vi "Read All Mixed Module Sizes.vi"(6 "MixedIO Mod Size Idxs":T14, 7 "R/W Case":T13, 8 "error in (no error)":errorcluster, 10 "Async in":T1, 11 "RSI Modules in":T2[](array[typedef]) {"Module Config Data"."Config Block Data Refs"."Data Reference" format="%.0x"; "CDOutput Data"."BD Refs"."Data Reference" format="%.0x"; "CDInput Data"."BD Refs"."Data Reference" format="%.0x"; "VS ref" format="%.0x"}) -> (0 "error out":errorcluster, 2 "Async out":T1, 3 "RSI Modules out":T2[](array[typedef]) {"Module Config Data"."Config Block Data Refs"."Data Reference" format="%.0x"; "CDOutput Data"."BD Refs"."Data Reference" format="%.0x"; "CDInput Data"."BD Refs"."Data Reference" format="%.0x"; "VS ref" format="%.0x"})   [LabVIEW 2020, in "SEECD Engine.lvlib"]
uses:
  SEECD Engine.lvlib
  Type Defs/Mod Size Indexes.ctl
  <vilib>/NI VeriStand/Custom Device API/Custom Device Item Ref.ctl
  <vilib>/NI VeriStand/Custom Device API/Custom Device API.lvlib
  <vilib>/NI VeriStand/Custom Device API/Data Reference.ctl
  <vilib>/NI VeriStand/Custom Device API/Block Data Reference.ctl
  Type Defs/Input Data.ctl
  Type Defs/Output Data.ctl
  Includes/Modules.lvlibp/RSI Module/Channel Type.ctl
  Includes/Modules.lvlibp/RSI Module/RSI Module.lvclass
  Includes/Modules.lvlibp/RSI Module/Module Models.ctl
  Type Defs/Module Config Data.ctl
  Type Defs/Mixed IO.ctl
  Type Defs/Open Module IOVs.ctl
  Type Defs/RSI Module Data.ctl
  Type Defs/RW Case.ctl
  Type Defs/Async Command.ctl
  Type Defs/Async State.ctl
  Type Defs/Async Status.ctl
  Type Defs/Async Data.ctl
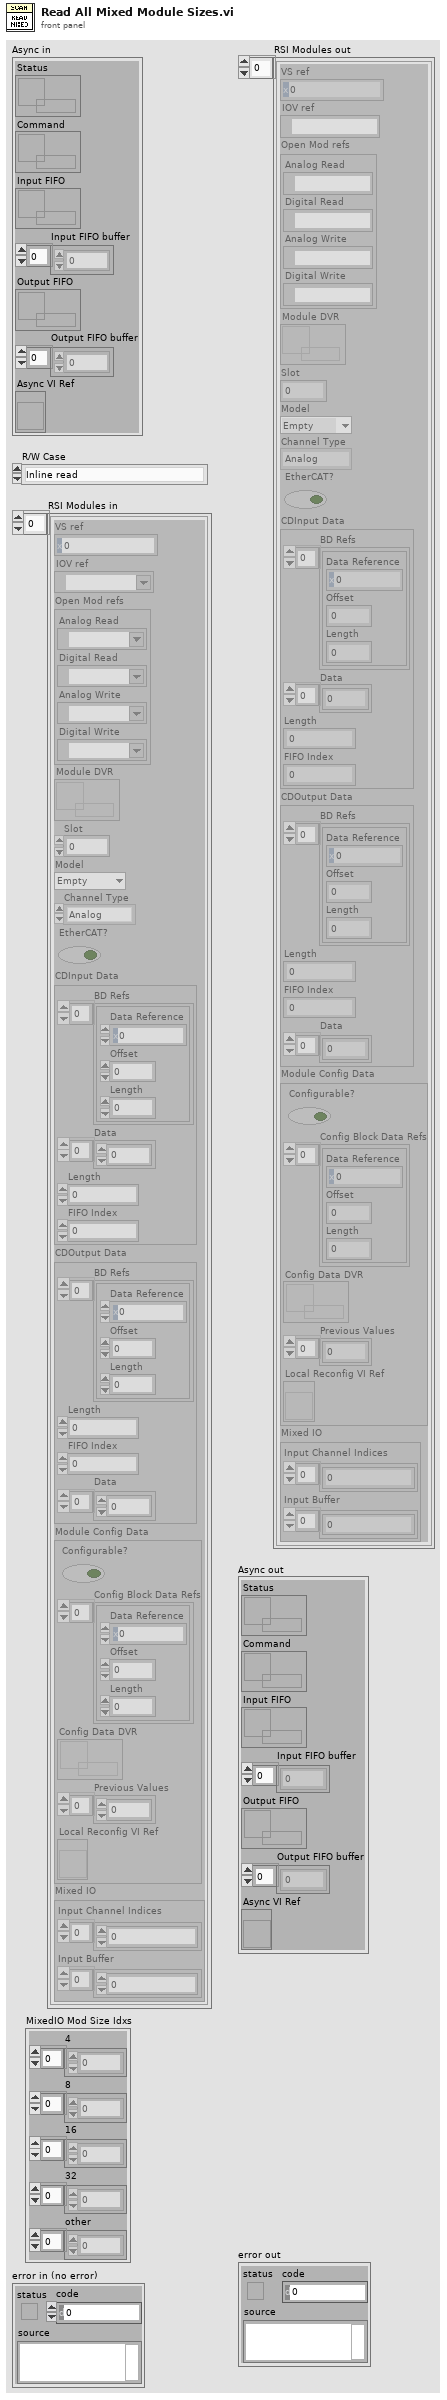
[diagram p1: front panel]
types:
  T1 = typedef "SEECD Engine.lvlib/Async Data.ctl" = cluster{"Status":refnum<queue>, "Command":refnum<queue>, "Input FIFO":refnum<k33>, "Input FIFO buffer":dbl[], "Output FIFO":refnum<k33>, "Output FIFO buffer":dbl[], "Async VI Ref":refnum<vi>}
  T2 = typedef "SEECD Engine.lvlib/RSI Module Data.ctl" = cluster{"VS ref":T3, "IOV ref":refnum<k21>, "Open Mod refs":T4, "Module DVR":refnum<data-value>, "Slot":u32, "Model":T5, "Channel Type":T6, "EtherCAT?":bool, "CDInput Data":T7, "CDOutput Data":T10, "Module Config Data":T11, "Mixed IO":T12}
  T3 = typedef "Custom Device API.lvlib/Custom Device Item Ref.ctl" = u64
  T4 = typedef "SEECD Engine.lvlib/Open Module IOVs.ctl" = cluster{"Analog Read":refnum<k21>, "Digital Read":refnum<k21>, "Analog Write":refnum<k21>, "Digital Write":refnum<k21>}
  T5 = typedef "Modules.lvlibp/RSI Module.lvclass/Module Models.ctl" = enum16{"Empty", "NI 9201", "NI 9203", "NI 9205", "NI 9206", "NI 9207", "NI 9208", "NI 9209", "NI 9210", "NI 9211", "NI 9212", "NI 9213", "NI 9214", "NI 9215", "NI 9216", "NI 9217", "NI 9219", "NI 9220", "NI 9221", "NI 9222", "NI 9223", "NI 9224", "NI 9225", "NI 9226", "NI 9227", "NI 9228", "NI 9229", "NI 9233", "NI 9234", "NI 9235", "NI 9236", "NI 9237", "NI 9239", "NI 9242", "NI 9244", "NI 9253", "NI 9263", "NI 9264", "NI 9265", "NI 9266", "NI 9269", "NI 9344", "NI 9350", "NI 9375", "NI 9401", "NI 9402", "NI 9403", "NI 9411", "NI 9421", "NI 9422", "NI 9423", "NI 9425", "NI 9426", "NI 9435", "NI 9436", "NI 9437", "NI 9472", "NI 9474", "NI 9475", "NI 9476", "NI 9477", "NI 9478", "NI 9481", "NI 9482", "NI 9485"}
  T6 = typedef "Modules.lvlibp/RSI Module.lvclass/Channel Type.ctl" = enum16{"Analog", "Digital"}
  T7 = typedef "SEECD Engine.lvlib/Input Data.ctl" = cluster{"BD Refs":T8[], "Data":dbl[], "Length":i32, "FIFO Index":i32}
  T8 = typedef "Custom Device API.lvlib/Block Data Reference.ctl" = cluster{"Data Reference":T9, "Offset":u64, "Length":u64}
  T9 = typedef "Custom Device API.lvlib/Data Reference.ctl" = i32
  T10 = typedef "SEECD Engine.lvlib/Output Data.ctl" = cluster{"BD Refs":T8[], "Length":i32, "FIFO Index":i32, "Data":dbl[]}
  T11 = typedef "SEECD Engine.lvlib/Module Config Data.ctl" = cluster{"Configurable?":bool, "Config Block Data Refs":T8[], "Config Data DVR":refnum<data-value>, "Previous Values":dbl[], "Local Reconfig VI Ref":refnum<vi>}
  T12 = typedef "SEECD Engine.lvlib/Mixed IO.ctl" = cluster{"Input Channel Indices":i32[], "Input Buffer":dbl[]}
  T13 = typedef "SEECD Engine.lvlib/RW Case.ctl" = enum16{"Inline read", "Inline write", "Async - Inline loop read", "Async - Inline loop write", "Async loop (read/write)"}
  T14 = typedef "SEECD Engine.lvlib/Mod Size Indexes.ctl" = cluster{"4":i32[], "8":i32[], "16":i32[], "32":i32[], "other":i32[]}
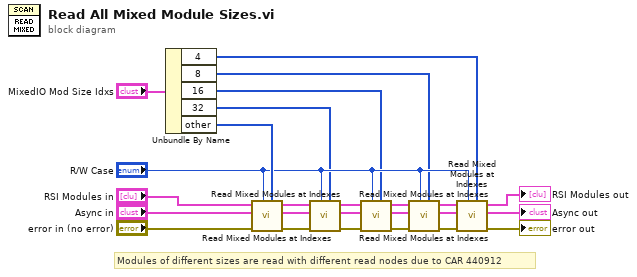
[diagram p0: block diagram]
diagram:
  # "Modules of different sizes are read with different read nodes due to CAR 440912"
  n1 = Unbundle By Name("MixedIO Mod Size Idxs") -> ("4"=w1:i32[], "8"=w2:i32[], "16"=w3:i32[], "32"=w4:i32[], "other"=w20:i32[])
  n2 = call "Read Mixed Modules at Indexes.vi"("Indexes"=w20, "R/W Case"="R/W Case", "error in (no error)"="error in (no error)", "Async in in"="Async in", "RSI Modules in in"="RSI Modules in") -> ("error out"=w25:errorcluster, "Async in out"=w17:T1, "RSI Modules in out"=w18:T2[])  [unwired: 4 in]
  n3 = call "Read Mixed Modules at Indexes.vi"("Indexes"=w4, "R/W Case"="R/W Case", "error in (no error)"=w25, "Async in in"=w17, "RSI Modules in in"=w18) -> ("error out"=w19:errorcluster, "Async in out"=w14:T1, "RSI Modules in out"=w15:T2[])  [unwired: 4 in]
  n4 = call "Read Mixed Modules at Indexes.vi"("Indexes"=w3, "R/W Case"="R/W Case", "error in (no error)"=w19, "Async in in"=w14, "RSI Modules in in"=w15) -> ("error out"=w16:errorcluster, "Async in out"=w11:T1, "RSI Modules in out"=w12:T2[])  [unwired: 4 in]
  n5 = call "Read Mixed Modules at Indexes.vi"("Indexes"=w2, "R/W Case"="R/W Case", "error in (no error)"=w16, "Async in in"=w11, "RSI Modules in in"=w12) -> ("error out"=w13:errorcluster, "Async in out"=w7:T1, "RSI Modules in out"=w9:T2[])  [unwired: 4 in]
  n6 = call "Read Mixed Modules at Indexes.vi"("Indexes"=w1, "R/W Case"="R/W Case", "error in (no error)"=w13, "Async in in"=w7, "RSI Modules in in"=w9) -> ("error out"=→"error out":errorcluster, "Async in out"=→"Async out":T1, "RSI Modules in out"=→"RSI Modules out":T2[])  [unwired: 4 in]
